vi "(Depricated) Differentiate Syringe Pressure.vi"(8 "error in (no error)":errorcluster, 10 "Syringe Pressure":dbl, 11 "cRIO Vacuum in":refnum<class "cRIO Vacuum.lvclass">) -> (0 "error out":errorcluster, 2 "d/dt":dbl, 3 "cRIO Vacuum out":refnum<class "cRIO Vacuum.lvclass">)   [LabVIEW 2015, in "cRIO-Carbondioxide.lvlib" / "CO2-Actor.lvlib" / "cRIO Vacuum.lvclass"]
uses:
  cRIO Vacuum.lvclass
  cRIO Vacuum.lvclass/cRIO Vacuum.ctl
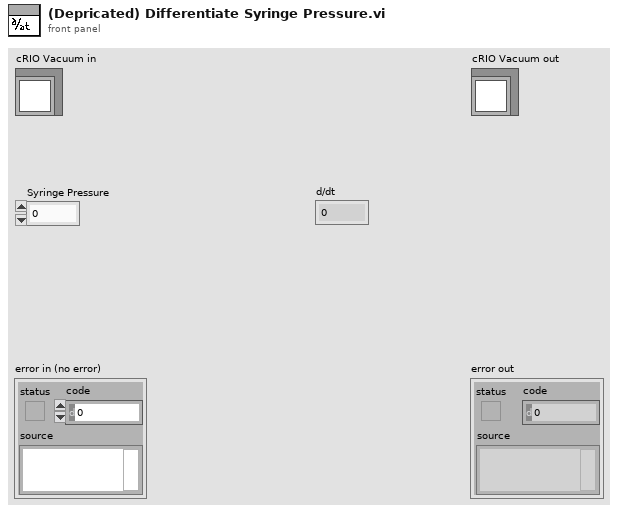
[diagram p1: front panel]
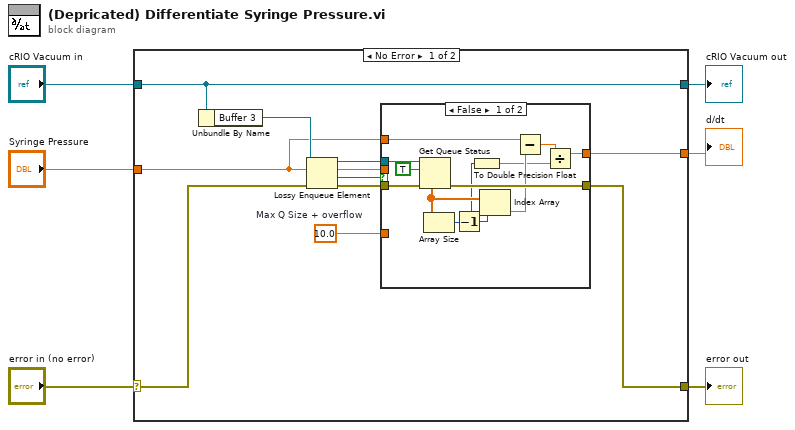
[diagram p0: block diagram]
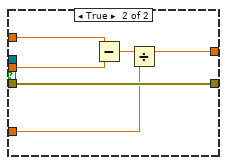
[diagram p2: hidden frame]
diagram:
  n1 = case shown="No Error" "error in (no error)" {
    selector: "error in (no error)" -> [w15 w36]
    tunnel: [w7 w36] -> w5
    tunnel: [w17 w37] -> w3
    tunnel: "cRIO Vacuum in" -> [w17 w37]
    tunnel: "Syringe Pressure" -> [w11 _]
    tunnel: [w9 _] -> w1
    frame No Error {
      w8 = 10.0  # Max Q Size + overflow
      n2 = Unbundle By Name(w17) -> ("Buffer 3"=w16:refnum<queue>)
      n3 = Lossy Enqueue Element(queue=w16, element=w11, error in (no error)=w15) -> (queue out=w12:refnum<queue>, overflow element=w10:dbl, overflow?=w13:bool, error out=w14:errorcluster)
      n4 = case shown="False" w13 {
        tunnel: w14 -> [w29 w32]
        tunnel: w12 -> [w28 _]
        tunnel: w11 -> [w22 w35]
        tunnel: w10 -> [_ w34]
        tunnel: [w21 w31] -> w9
        tunnel: [w24 w32] -> w7
        tunnel: w8 -> [_ w30]
        frame False {
          n5 = Get Queue Status(queue=w28, return elements? (F)=TRUE, error in (no error)=w29) -> (error out=w24:errorcluster, elements=w26:dbl[])  [unwired: 6 out]
          n6 = Array Size(array=w26) -> (size(s)=w20:i32)
          n7 = Decrement(x=w20) -> (x-1=w25:i32)
          n8 = To Double Precision Float(number=w20) -> (double precision float=w18:dbl)
          n9 = Index Array(array=w26, index=w25) -> (element=w23:dbl)
          n10 = Subtract(x=w22, y=w23) -> (x-y=w19:dbl)
          n11 = Divide(x=w19, y=w18) -> (x/y=w21:dbl)
        }
        frame True {
          n12 = Subtract(x=w35, y=w34) -> (x-y=w33:dbl)
          n13 = Divide(x=w33, y=w30) -> (x/y=w31:dbl)
        }
      }
    }
    frame Error {
    }
  }
  "error out" <- w5
  "cRIO Vacuum out" <- w3
  "d/dt" <- w1
